vi "DIAdem Scripts Folder.vi"(3 "Relative Path (\"\" - Folder)":string) -> (1 "Scripts Folder":path)   [LabVIEW 2011]
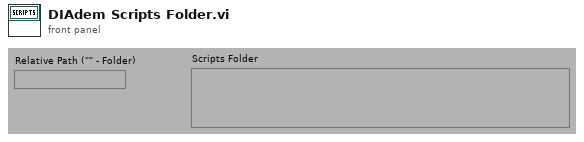
[diagram p1: front panel]
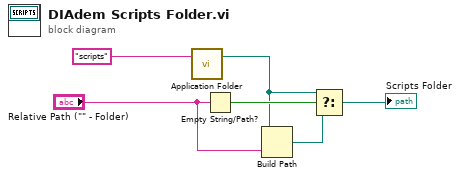
[diagram p0: block diagram]
diagram:
  n1 = call "Application Folder.vi"("Relative Path (\"\" - Folder)"="scripts" ("name or relative path")) -> ("Application Folder"=w1:path)  [unwired: 2 in]
  n2 = Empty String/Path?(string/path="Relative Path (\"\" - Folder)") -> (empty?=w5:bool)
  n3 = Build Path(base path=w1, name or relative path="Relative Path (\"\" - Folder)") -> (appended path=w3:path)
  n4 = Select(t=w1, s=w5, f=w3) -> (s? t:f=→"Scripts Folder":path)
